vi "ArrayAsIntegers.vi"(8 "error in (no error)":errorcluster, 11 "Array Parameter":string="\n      <array>\n  <data>\r<value><double>0.000000</double></value>\r<value><double>1.175571</double></value>\r<value><double>1.902113</double></value>\r<value><double>1.902113</double></value>\r<value><double>1.175571</double></value>\r<value><double>0.000000</double></value>\r<value><double>-1.175571</double></value>\r<value><double>-1.902113</double></value>\r<value><double>-1.902113</double></value>\r<value><double>-1.175571</double></value>\r<value><double>0.000000</double></value>\r<value><double>1.175571</double></value>\r<value><double>1.902113</double></value>\r<value><double>1.902113</double></value>\r<value><double>1.175571</double></value>\r<value><double>0.000000</double></value>\r<value><double>-1.175571</double></value>\r<value><double>-1.902113</double></value>\r<value><double>-1.902113</double></value>\r<value><double>-1.175571</double></value>\r<value><double>0.000000</double></value>\r<value><double>1.175571</double></value>\r<value><double>1.902113</double></value>\r<value><double>1.902113</double></value>\r<value><double>1.175571</double></value>\r<value><double>0.000000</double></value>\r<value><double>-1.175571</double></value>\r<value><double>-1.902113</double></value>\r<value><double>-1.902113</double></value>\r<value><double>-1.175571</double></value>\r<value><double>0.000000</double></value>\r<value><double>1.175571</double></value>\r<value><double>1.902113</double></value>\r<value><double>1.902113</double></value>\r<value><double>1.175571</double></value>\r<value><double>0.000000</double></value>\r<value><double>-1.175571</double></value>\r<value><double>-1.902113</double></value>\r<value><double>-1.902113</double></value>\r<value><double>-1.175571</double></value>\r<value><double>0.000000</double></value>\r<value><double>1.175571</double></value>\r<value><double>1.902113</double></value>\r<value><double>1.902113</double></value>\r<value><double>1.175571</double></value>\r<value><double>0.000000</double></value>\r<value><double>-1.175571</double></value>\r<value><double>-1.902113</double></value>\r<value><double>-1.902113</double></value>\r<value><double>-1.175571</double></value>\r<value><double>0.000000</double></value>\r<value><double>1.175571</double></value>\r<value><double>1.902113</double></value>\r<value><double>1.902113</double></value>\r<value><double>1.175571</double></value>\r<value><double>0.000000</double></value>\r<value><double>-1.175571</double></value>\r<value><double>-1.902113</double></value>\r<value><double>-1.902113</double></value>\r<value><double>-1.175571</double></value>\r<value><double>0.000000</double></value>\r<value><double>1.175571</double></value>\r<value><double>1.902113</double></value>\r<value><double>1.902113</double></value>\r<value><double>1.175571</double></value>\r<value><double>0.000000</double></value>\r<value><double>-1.175571</double></value>\r<value><double>-1.902113</double></value>\r<value><double>-1.902113</double></value>\r<value><double>-1.175571</double></value>\r<value><double>0.000000</double></value>\r<value><double>1.175571</double></value>\r<value><double>1.902113</double></value>\r<value><double>1.902113</double></value>\r<value><double>1.175571</double></value>\r<value><double>0.000000</double></value>\r<value><double>-1.175571</double></value>\r<value><double>-1.902113</double></value>\r<value><double>-1.902113</double></value>\r<value><double>-1.175571</double></value>\r<value><double>0.000000</double></value>\r<value><double>1.175571</double></value>\r<value><double>1.902113</double></value>\r<value><double>1.902113</double></value>\r<value><double>1.175571</double></value>\r<value><double>0.000000</double></value>\r<value><double>-1.175571</double></value>\r<value><double>-1.902113</double></value>\r<value><double>-1.902113</double></value>\r<value><double>-1.175571</double></value>\r<value><double>0.000000</double></value>\r<value><double>1.175571</double></value>\r<value><double>1.902113</double></value>\r<value><double>1.902113</double></value>\r<value><double>1.175571</double></value>\r<value><double>0.000000</double></value>\r<value><double>-1.175571</double></value>\r<value><double>-1.902113</double></value>\r<value><double>-1.902113</double></value>\r<value><double>-1.175571</double></value>\r<value><double>0.000000</double></value>\r<value><double>1.175571</double></value>\r<value><double>1.902113</double></value>\r<value><double>1.902113</double></value>\r<value><double>1.175571</double></value>\r<value><double>0.000000</double></value>\r<value><double>-1.175571</double></value>\r<value><double>-1.902113</double></value>\r<value><double>-1.902113</double></value>\r<value><double>-1.175571</double></value>\r<value><double>0.000000</double></value>\r<value><double>1.175571</double></value>\r<value><double>1.902113</double></value>\r<value><double>1.902113</double></value>\r<value><double>1.175571</double></value>\r<value><double>0.000000</double></value>\r<value><double>-1.175571</double></value>\r<value><double>-1.902113</double></value>\r<value><double>-1.902113</double></value>\r<value><double>-1.175571</double></value>\r<value><double>0.000000</double></value>\r<value><double>1.175571</double></value>\r<value><double>1.902113</double></value>\r<value><double>1.902113</double></value>\r<value><double>1.175571</double></value>\r<value><double>0.000000</double></value>\r<value><double>-1.175571</double></value>\r<value><double>-1.902113</double></value>\n  </data>\n</array>\n    ") -> (0 "error out":errorcluster, 3 "ArrayAsInts":i32[](array[numeric]))   [LabVIEW 2009]
doc: "Convert an XML-RPC formatted array of integers to a LV array of integers"
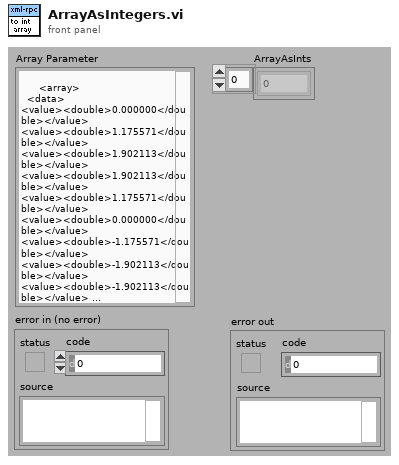
[diagram p1: front panel]
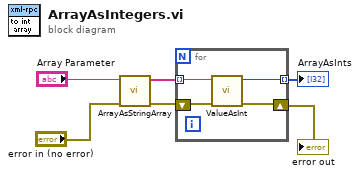
[diagram p0: block diagram]
diagram:
  n1 = call "ArrayAsStringArray.vi"("error in (no error)"="error in (no error)", "Array Parameter"="Array Parameter") -> ("error out"=w3:errorcluster, "ArrayAsValues"=w4:string[])  [unwired: 8 in]
  n2 = for {
    tunnel: w4 -> [w10] mode=indexing
    shift-right: [w8] -> w1
    shift-left: w3 -> [w9]
    tunnel: [w7] -> w2 mode=indexing
    n3 = call "ValueAsInt.vi"("error in (no error)"=w9, "Parameter"=w10) -> ("error out"=w8:errorcluster, "value"=w7:i32)  [unwired: 8 in]
  }
  "ArrayAsInts" <- w2
  "error out" <- w1
